vi "Fibonacci.vi"() -> ()   [LabVIEW 2018]
panel:
  out "Boolean":bool
  in  "stop":bool
  out "Fibonacci":string
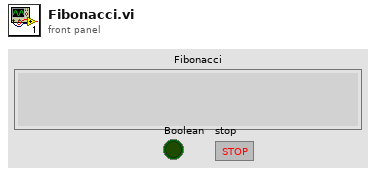
[diagram p1: front panel]
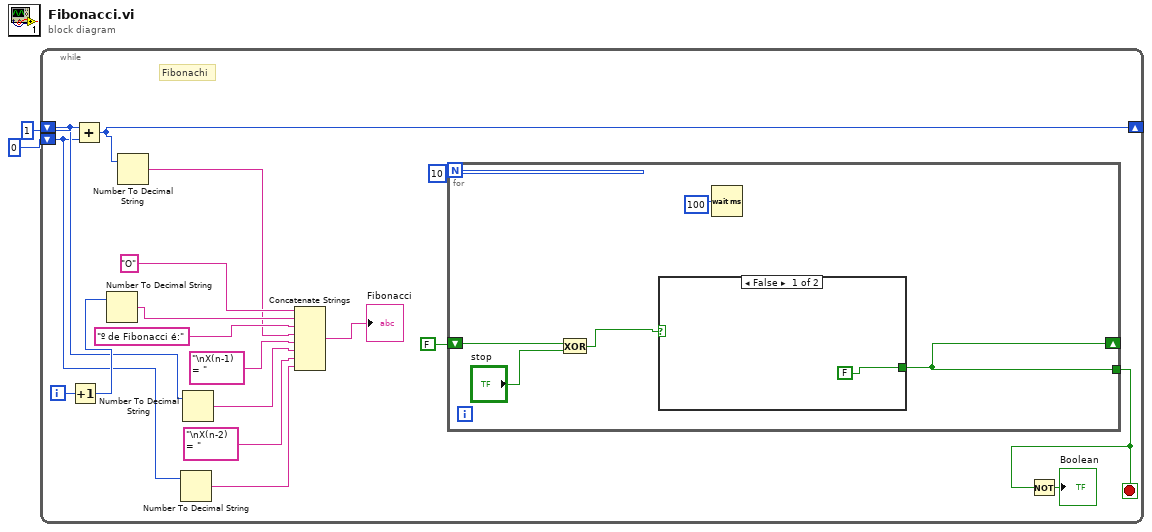
[diagram p0: block diagram]
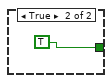
[diagram p2: hidden frame]
diagram:
  n1 = while {
    shift-right: [w18] -> _
    shift-left: 1 -> [w7]
    shift-left: 0 -> [w6]
    i -> [w20]
    stop <- w3 stop-if-true
    # "Fibonachi"
    n2 = Increment(x=w20) -> (x+1=w19:i32)
    n3 = Add(x=w7, y=w6) -> (x+y=w18:i32)
    n4 = Number To Decimal String(number=w19) -> (decimal integer string=w16:string)  [unwired: 1 in]
    n5 = Number To Decimal String(number=w18) -> (decimal integer string=w14:string)  [unwired: 1 in]
    n6 = Number To Decimal String(number=w6) -> (decimal integer string=w8:string)  [unwired: 1 in]
    n7 = Number To Decimal String(number=w7) -> (decimal integer string=w10:string)  [unwired: 1 in]
    n8 = Concatenate Strings("O", w16, "º de Fibonacci é:", w14, "\nX(n-1) = ", w10, "\nX(n-2) = ", w8) -> (→"Fibonacci":string)
    n9 = for {
      N: 10 -> [_]
      tunnel: [w24] -> w3
      shift-right: [w24] -> _
      shift-left: FALSE -> [w22]
      n10 = Exclusive Or(1:"stop", 2:w22) -> (0:w21:bool)
      n11 = case shown="False" w21 {
        tunnel: [FALSE TRUE] -> w24
        frame False {
        }
        frame True {
        }
      }
      n12 = Wait (ms)(milliseconds to wait=u32 100) -> ()  [unwired: 1 out]
    }
    n13 = Not(x=w3) -> (.not. x?=→"Boolean":bool)
  }
